vi "Get Channel.vi"(8 "error in (no error)":errorcluster, 10 "Channel Name":string, 11 "CIFChannelMng in":refnum<class "CIFChannelMng.lvclass">) -> (0 "error out":errorcluster, 2 "Channel":refnum<class "CIFChannels.lvclass">, 3 "CIFChannelMng out":refnum<class "CIFChannelMng.lvclass">)   [LabVIEW 2021, in "CIFChannelMng.lvclass"]
uses:
  CIFChannelMng.lvclass
  CIFChannels/CIFChannels.lvclass
  CIFChannelMng.lvclass/CIFChannelMng.ctl
  CIFClocks/Typedef/Errors.ctl
  CIFCore/Common/Utilities/Append Error Location.vi
  CIFCore/Common/CIFCoreCommon.lvlib
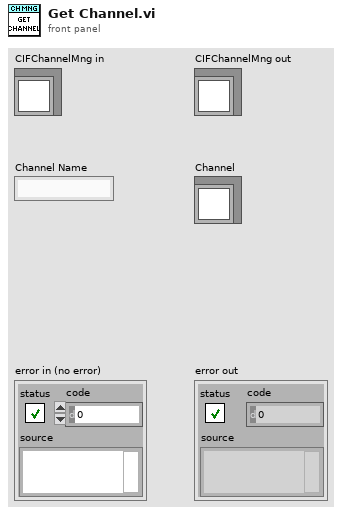
[diagram p1: front panel]
types:
  T1 = typedef "CIFCoreCommon.lvlib/Errors.ctl" = enum16{"Invalid Clock ID", "Long Sleep", "gRPC Server Not Found", "Config Parse", "Timestamp Wrap", "Delayed Execution", "Duplicate Channel", "Missing Channel", "Incorrect Type", "Unregistered Enum"}
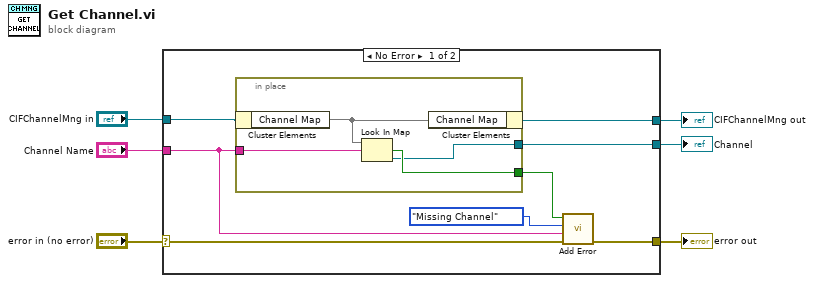
[diagram p0: block diagram]
diagram:
  n1 = case shown="No Error" "error in (no error)" {
    selector: "error in (no error)" -> [w8 w20]
    tunnel: [w11 w20] -> w6
    tunnel: [w14 w19] -> w5
    tunnel: "CIFChannelMng in" -> [w9 w19]
    tunnel: "Channel Name" -> [w7 _]
    tunnel: [w10 _] -> w4
    frame No Error {
      n2 = in-place {
        in-place-border: w7 -> [w18]
        in-place-border: [w17] -> w13
        in-place-border: [w16] -> w10
        n3 = in-place-cluster #1(w9) -> ("Channel Map"=w15:map{string, refnum<class "CIFChannels.lvclass">})
        n4 = Look In Map(map=w15, key=w18) -> (key not found?=w17:bool, value=w16:refnum<class "CIFChannels.lvclass">)  [unwired: 1 in]
        n5 = in-place-cluster #1("Channel Map"=w15) -> (w14:refnum<class "CIFChannelMng.lvclass">)
      }
      n6 = call "Add Error.vi"("error in (no error)"=w8, "String to Append"=w7, "Error"=Errors."Missing Channel", "Insert Error"=w13) -> ("error out"=w11:errorcluster)  [unwired: 7 in]
    }
    frame Error {
    }
  }
  "error out" <- w6
  "CIFChannelMng out" <- w5
  "Channel" <- w4
